vi "From Minimal Cluster.vi"(8 "error in (no error)":errorcluster, 9 "Receiving Queue":refnum<queue>, 10 "Log Directory":path, 11 "Minimal Controller Cluster":T1) -> (0 "error out":errorcluster, 3 "Generic Controller out":refnum<class "Generic Plugin.lvclass">)   [LabVIEW 2020, in "Generic Plugin.lvclass"]
doc: "Similar VI to Initialize Controller, but most parameters are now read from a minimal cluster."
uses:
  Generic Plugin.lvclass
  Minimal Controller Cluster.ctl
  <userlib>/Dynamic Reentrant/Type Defs/Message.ctl
  Controller Type.ctl
  Generic Plugin.lvclass/Generic Plugin.ctl
  <userlib>/Dynamic Reentrant/Dynamic Reentrant.lvlib
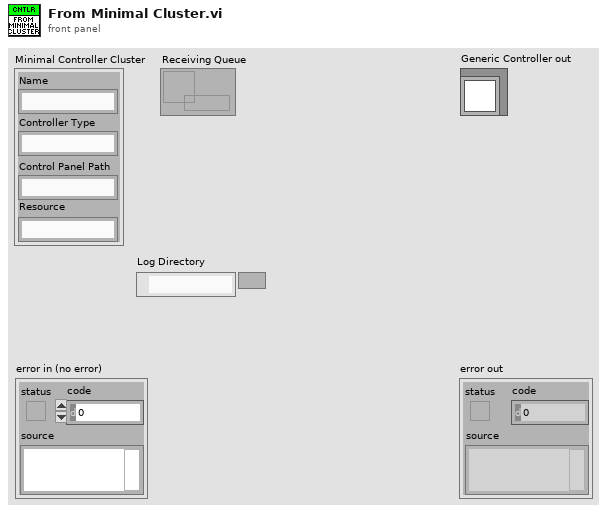
[diagram p1: front panel]
types:
  T1 = typedef "Generic Plugin.lvclass/Minimal Controller Cluster.ctl" = cluster{"Name":string, "Controller Type":string, "Control Panel Path":string, "Resource":string}
  T2 = typedef "Generic Plugin.lvclass/Controller Type.ctl" = enum16{"Invalid", "Temperature Controller", "Pump Controller", "Generic Optimizer", "LC Parser"}
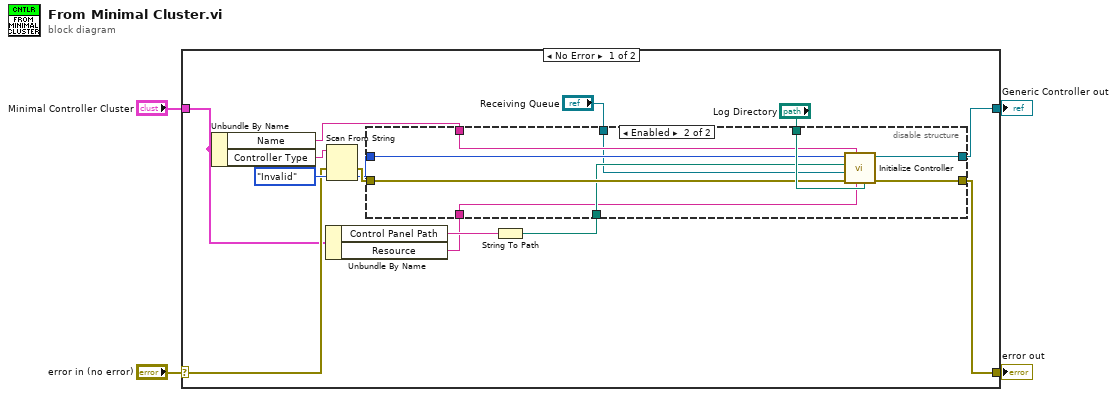
[diagram p0: block diagram]
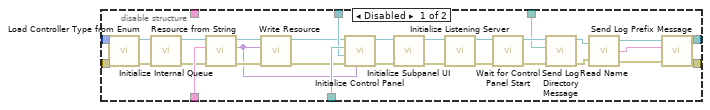
[diagram p2: hidden frame]
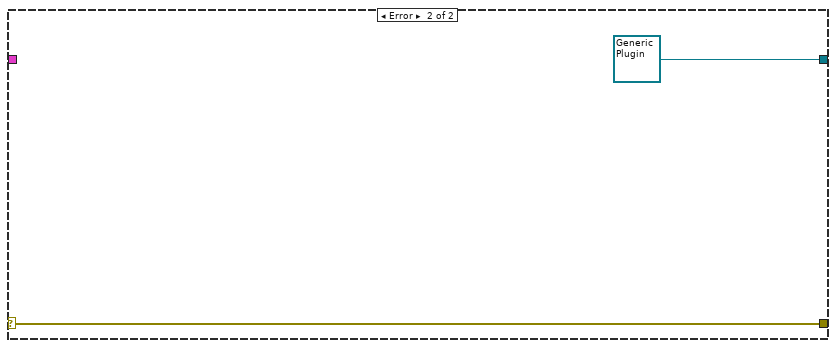
[diagram p3: hidden frame]
diagram:
  n1 = case shown="No Error" "error in (no error)" {
    selector: "error in (no error)" -> [w14 w59]
    tunnel: [w9 w59] -> w3
    tunnel: [w8 refnum<class "Generic Plugin.lvclass"> refnum ("Generic Controller out")] -> w2
    tunnel: "Minimal Controller Cluster" -> [w13 _]
    frame No Error {
      n2 = Unbundle By Name(w13) -> ("Name"=w5:string, "Controller Type"=w15:string)
      n3 = Unbundle By Name(w13) -> ("Control Panel Path"=w12:string, "Resource"=w10:string)
      n4 = Scan From String(input string=w15, error in=w14, default 1=Controller_Type."Invalid" ("Controller Type")) -> (error out=w18:errorcluster, output 1=w16:T2)  [unwired: 2 in, 2 out]
      n5 = String To Path(string=w12) -> (path=w11:path)
      n6 = disable-structure shown="Enabled" {
        disable-tunnel: w18 -> [w48 w52]
        disable-tunnel: w16 -> [w39 w53]
        disable-tunnel: w11 -> [w38 w51]
        disable-tunnel: w10 -> [w36 w49]
        disable-tunnel: [w31 w56] -> w9
        disable-tunnel: [w30 w57] -> w8
        disable-tunnel: "Log Directory" -> [w29 w55]
        disable-tunnel: "Receiving Queue" -> [w28 w50]
        disable-tunnel: w5 -> [_ w54]
        frame Disabled {
          n7 = call "Load Controller Type from Enum.vi"("error in (no error)"=w48, "Controller Type"=w39) -> ("error out"=w40:errorcluster, "controller out"=w47:refnum<class "Generic Plugin.lvclass">)  [unwired: 8 in]
          n8 = call "Initialize Internal Queue.vi"("error in (no error)"=w40, "Generic Controller in"=w47) -> ("error out"=w35:errorcluster, "Generic Controller out"=w37:refnum<class "Generic Plugin.lvclass">)  [unwired: 8 in]
          n9 = call-dynamic "Resource from String.vi"("error in (no error)"=w35, "Resource from String"=w36, "Generic Controller in"=w37) -> ("error out"=w34:errorcluster, "Resource as Variant"=w19:variant, "Generic Controller out"=w21:refnum<class "Generic Plugin.lvclass">)  [unwired: 6 in]
          n10 = call-dynamic "Write Resource.vi"("error in (no error)"=w34, "Resource"=w19, "Generic Controller in"=w21) -> ("error out"=w22:errorcluster, "Generic Controller out"=w20:refnum<class "Generic Plugin.lvclass">)  [unwired: 7 in]
          n11 = call "Initialize Control Panel.vi"("Resource"=w19, "error in (no error)"=w22, "Receiving Queue"=w28, "Control Panel Path"=w38, "Generic Controller in"=w20) -> ("error out"=w43:errorcluster, "Generic Controller out"=w42:refnum<class "Generic Plugin.lvclass">)  [unwired: 5 in]
          n12 = call "Initialize Subpanel UI.vi"("error in (no error)"=w43, "Plugin in"=w42) -> ("error out"=w41:errorcluster, "Plugin out"=w45:refnum<class "Generic Plugin.lvclass">)  [unwired: 7 in, 1 out]
          n13 = call "Initialize Listening Server.vi"("error in (no error)"=w41, "Generic Controller in"=w45) -> ("error out"=w44:errorcluster, "Generic Controller out"=w46:refnum<class "Generic Plugin.lvclass">)  [unwired: 7 in, 1 out]
          n14 = call "Wait for Control Panel Start.vi"("error in (no error)"=w44, "Generic Controller in"=w46) -> ("error out"=w33:errorcluster, "Generic Controller out"=w32:refnum<class "Generic Plugin.lvclass">)  [unwired: 8 in]
          n15 = call "Send Log Directory Message.vi"("error in (no error)"=w33, "Log Directory"=w29, "Generic Controller in"=w32) -> ("error out"=w27:errorcluster, "Generic Controller out"=w25:refnum<class "Generic Plugin.lvclass">)  [unwired: 7 in]
          n16 = call "Read Name.vi"("controller in"=w25, "error in (no error)"=w27) -> ("controller out"=w24:refnum<class "Generic Plugin.lvclass">, "Name"=w23:string, "error out"=w26:errorcluster)
          n17 = call "Send Log Prefix Message.vi"("error in (no error)"=w26, "Log Prefix"=w23, "Generic Controller in"=w24) -> ("error out"=w31:errorcluster, "Generic Controller out"=w30:refnum<class "Generic Plugin.lvclass">)  [unwired: 7 in]
        }
        frame Enabled {
          n18 = call "Initialize Controller.vi"("Log Directory"=w55, "Resource"=w49, "Instance Name"=w54, "error in (no error)"=w52, "Receiving Queue"=w50, "Control Panel Path"=w51, "Controller Type"=w53) -> ("error out"=w56:errorcluster, "Generic Controller out"=w57:refnum<class "Generic Plugin.lvclass">)  [unwired: 3 in]
        }
      }
    }
    frame Error {
    }
  }
  "error out" <- w3
  "Generic Controller out" <- w2
